vi "Do.vi"(8 "error in (no error)":errorcluster, 10 "Actor in":refnum<class "Actor.lvclass">, 11 "TDMS Cleanup Msg in":refnum<class "TDMS Cleanup Msg.lvclass">) -> (0 "error out":errorcluster, 2 "Actor out":refnum<class "Actor.lvclass">)   [LabVIEW 2020, in "Logging.lvlib" / "TDMS Cleanup Msg.lvclass"]
doc: "(<B>Filename</B>: Actor Framework.lvlib:Message.lvclass:Do.vi)\n\nDefines what a message does when it is received by an actor. Generally, a message instructs an actor to invoke one of its methods. By default, this method does nothing. A child class must override it to define behavior. Create a child class by using the Actor Framework Message Maker dialog box."
uses:
  TDMS Cleanup Msg.lvclass
  <vilib>/ActorFramework/Actor/Actor.lvclass
  Logging/Logging.lvclass
  C:/Program Files/National Instruments/LabVIEW 2020/vi.lib/ActorFramework/Actor/Actor.lvclass
  TDMS Cleanup Msg.lvclass/TDMS Cleanup Msg.ctl
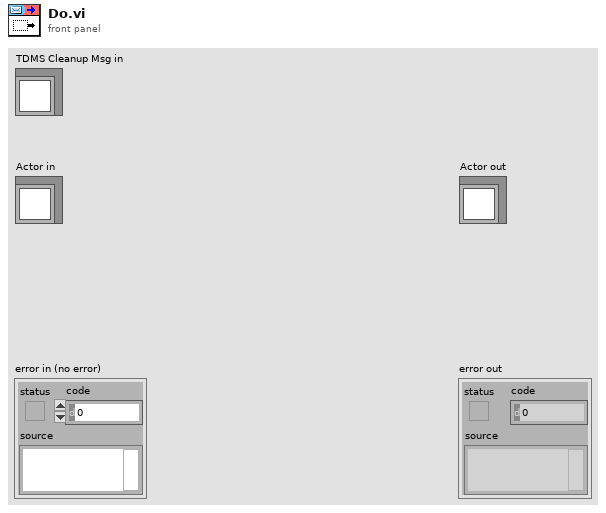
[diagram p1: front panel]
types:
  T1 = typedef "Task selection df.ctl" = cluster{"Task Type Select":enum32{"Frequency Task", "Scanning Task"}, "Input Select Type":enum32{"Force Input", "Movement Input"}, "Collect EMG?":bool, "Collect acceleration?":bool, "EMG Rate":u16, "Acceleration Rate":u16}
  T2 = typedef "Task info df.ctl" = cluster{"Number of Trials":u8, "Sampling Rate (Hz)":u16, "Trial Duration (s)":u8, "Adjusted MVC (N)":dbl, "R Phase":i32, "L Phase":i32, "L Pattern":u8, "R Pattern":u8, "Time Between Trials (s)":u8, "Lissajous Speed":u16}
  T3 = typedef "Automate df.ctl" = cluster{"Automate?":bool, "Num Parabs":u16, "Patterns Array":u8[][], "Phase Array":i32[][]}
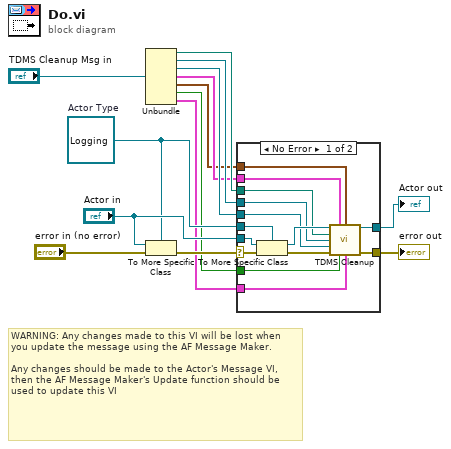
[diagram p0: block diagram]
diagram:
  w9 = refnum<class "Logging.lvclass"> refnum  # Actor Type
  # "WARNING: Any changes made to this VI will be lost when you update the message using the AF Message Maker.\n\nAny changes should be made to the Actor's Message VI, then the AF Message Maker's Update function should be used to update this VI"
  n1 = Unbundle("TDMS Cleanup Msg in") -> (w8:path, w7:refnum<k34>, w6:refnum<k34>, w5:T1, w4:T2, w3:bool, w2:T3)
  n2 = To More Specific Class(target class=w9, reference="Actor in", error in="error in (no error)") -> (error out=w13:errorcluster)  [unwired: 1 out]
  n3 = case shown="No Error" w13 {
    selector: w13 -> [w28 w30]
    tunnel: [w23 w30] -> w12
    tunnel: [w22 w29] -> w11
    tunnel: "Actor in" -> [w27 w29]
    tunnel: w9 -> [w26 _]
    tunnel: w8 -> [w21 _]
    tunnel: w7 -> [w20 _]
    tunnel: w6 -> [w19 _]
    tunnel: w5 -> [w18 _]
    tunnel: w4 -> [w17 _]
    tunnel: w3 -> [w16 _]
    tunnel: w2 -> [w15 _]
    frame No Error {
      n4 = To More Specific Class ("Actor Cast")(target class=w26, reference=w27, error in=w28) -> (specific class reference=w25:refnum<class "Logging.lvclass">, error out=w24:errorcluster)
      n5 = call "TDMS Cleanup.vi"("Logging in"=w25, "Task Selection"=w18, "Task info"=w17, "TDMS File"=w21, "Accel TDMS File"=w20, "Force TDMS File"=w19, "error in (no error)"=w24, "Movement?"=w16, "Auto Clust"=w15) -> ("Logging out"=w22:refnum<class "Logging.lvclass">, "error out"=w23:errorcluster)  [unwired: 5 in]
    }
    frame Error {
    }
  }
  "error out" <- w12
  "Actor out" <- w11
